vi "Test App Trigger Broadcast of Owned Process.vi"(8 "error in (no error)":errorcluster, 11 "Application Test in":refnum<class "Application Test.lvclass">) -> (0 "error out":errorcluster, 3 "Application Test out":refnum<class "Application Test.lvclass">)   [LabVIEW 2020, in "Application Test.lvclass"]
uses:
  Application Test.lvclass
  C:/Program Files (x86)/National Instruments/LabVIEW 2020/vi.lib/Asteme/LUnit/Test Case.lvclass
  Framework/Process/Process.lvclass
  Framework/Process/Process.lvclass/Process.ctl
  Framework/Application/Application.lvclass/Application.ctl
  <vilib>/Asteme/LUnit/Test Case.lvclass/Test Case.ctl
  <vilib>/Asteme/LUnit/LUnit Assertion Result.lvclass/LUnit Assertion Result.ctl
  Framework/Application/Private/Add Process to Map.vi
  Framework/Application/Private/Start Idle Processes if Running.vi
  Framework/Process/Protected/Messaging/Enqueue Message.vi
  Framework/Process/Public/Lifecycle/Get Lifecycle State.vi
  Framework/Process/Protected/SubVIs/Set Context.vi
  Framework/Process/Private/SubVIs/Wait for finish.vi
  Framework/Process/Private/SubVIs/Set Lifecycle State.vi
  <vilib>/Asteme/LUnit/Palette/Fail.vi
  <vilib>/Asteme/LUnit/Palette/Pass.vi
  <vilib>/Asteme/LUnit/Set Assertion Type.vi
  <vilib>/Utility/error.llb/Clear Errors.vi
  Framework/Process/Public/Lifecycle/Leave Process Loop.vi
  <vilib>/Asteme/LUnit/Add test result.vi
  <vilib>/Asteme/LUnit/LUnit Write Passed.vi
  <vilib>/Asteme/LUnit/LUnit Get Test Case.vi
  <vilib>/Asteme/LUnit/Assertion Result/LUnit Get Test Name.vi
  <vilib>/Asteme/LUnit/LUnit Write Message.vi
  <vilib>/Asteme/LUnit/LUnit Write Description.vi
  <vilib>/Asteme/LUnit/LUnit Write Assertion Type.vi
  <vilib>/Asteme/LUnit/Read Test Case Name.vi
  Framework/Application/Application.lvclass
  C:/Users/anton/Documents/GitHub/Triarc-Framework/source/Framework/Process/Process.lvclass
  <vilib>/Utility/error.llb/Error Cluster From Error Code.vi
  Framework/Application/Private/Update Context for Owned Processes.vi
  <vilib>/Asteme/LUnit/LUnit Assertion Result.lvclass
  <vilib>/Asteme/LUnit/Test Case.lvclass
  Support/Framework Test Support.lvlib
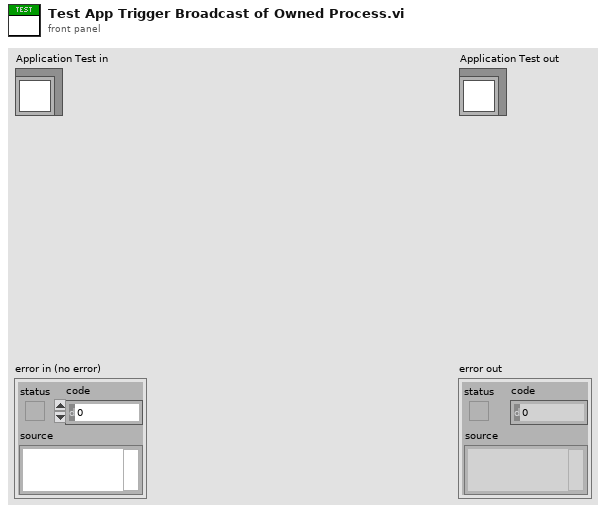
[diagram p1: front panel]
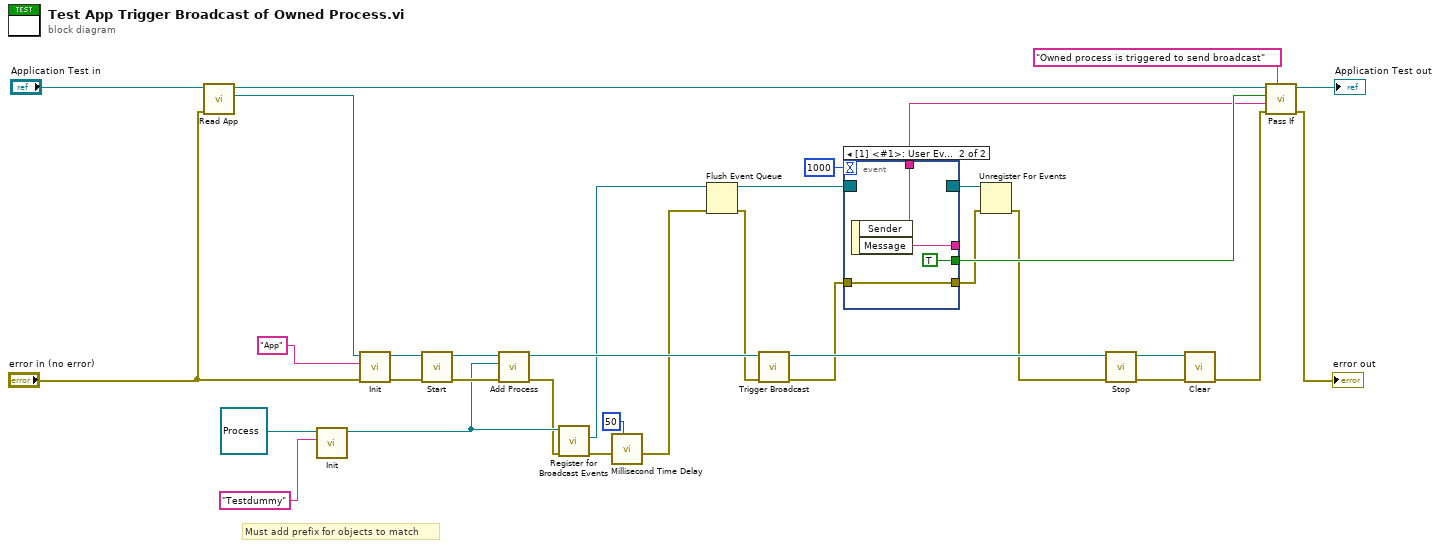
[diagram p0: block diagram]
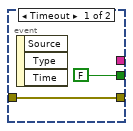
[diagram p2: hidden frame]
diagram:
  # "Must add prefix for objects to match"
  n1 = call "Read App.vi"("error in (no error)"="error in (no error)", "Application Test In"="Application Test in") -> ("App out"=w33:refnum<class "Application.lvclass">, "Application Test Out"=w34:refnum<class "Application Test.lvclass">)  [unwired: 7 in, 1 out]
  n2 = call-dynamic "Init.vi"("Name"="Testdummy", "Process In"=refnum<class "Process.lvclass"> refnum ("Process.lvclass")) -> ("Process Out"=w21:refnum<class "Process.lvclass">)  [unwired: 8 in, 1 out]
  n3 = call-dynamic "Init.vi"("error in (no error)"="error in (no error)", "Name"="App", "Process In"=w33) -> ("error out"=w31:errorcluster, "Process Out"=w32:refnum<class "Application.lvclass">)  [unwired: 7 in]
  n4 = call "Start.vi"("error in (no error)"=w31, "Process In"=w32) -> ("error out"=w29:errorcluster, "Process Out"=w22:refnum<class "Application.lvclass">)  [unwired: 8 in]
  n5 = call "Add Process.vi"("error in (no error)"=w29, "Process"=w21, "Rig In"=w22) -> ("error out"=w20:errorcluster, "Rig Out"=w19:refnum<class "Application.lvclass">)  [unwired: 7 in]
  n6 = call "Register for Broadcast Events.vi"("error in (no error)"=w20, "Process In"=w21) -> ("error out"=w5:errorcluster, "Event Registration Refnum Out"=w8:refnum<event-registration>)  [unwired: 7 in, 1 out]
  n7 = call "Millisecond Time Delay.vi"("milliseconds to wait"=u32 50, "error in (no error)"=w5) -> ("error out"=w4:errorcluster)  [unwired: 7 in]
  n8 = Flush Event Queue(0:w8, 3:w4) -> (8:w7:refnum<event-registration>, 11:w6:errorcluster)  [unwired: 4 in, 1 out]
  n9 = call "Trigger Broadcast.vi"("error in (no error)"=w6, "Process in"=w19) -> ("error out"=w10:errorcluster, "Process out"=w18:refnum<class "Application.lvclass">)  [unwired: 8 in]
  n10 = event shown="[1] <#1>: User Event" {
    selector: w7 -> [_ _]
    dyn-events: [_ _] -> w17
    timeout: 1000 -> [_ _]
    tunnel: [FALSE TRUE] -> w15
    tunnel: [w35 w39] -> w2
    tunnel: w10 -> [w35 w39]
    tunnel: [_ w38] -> w9
    tunnel: [_ w37] -> _
    event Timeout {
      n11 = event-data() -> ()  [unwired: 1 in, 3 out]
    }
    event User Event {
      n12 = event-data() -> ("Sender"=w38:string, "Message"=w37:string)  [unwired: 1 in]
    }
  }
  n13 = Unregister For Events(event registration refnum=w17, error in=w2) -> (error out=w1:errorcluster)
  n14 = call "Stop.vi"("error in (no error)"=w1, "Process In"=w18) -> ("error out"=w27:errorcluster, "Process Out"=w30:refnum<class "Application.lvclass">)  [unwired: 7 in, 1 out]
  n15 = call-dynamic "Clear.vi"("error in (no error)"=w27, "Application In"=w30) -> ("error out"=w14:errorcluster)  [unwired: 9 in]
  n16 = call <vilib>:"Pass If.vi"("Description"="Owned process is triggered to send broadcast", "error in (no error)"=w14, "Message"=w9, "Pass?"=w15, "Test Case In"=w34) -> ("error out"=→"error out":errorcluster, "Test Case Out"=→"Application Test out":refnum<class "Application Test.lvclass">)  [unwired: 5 in]
